vi "Controller FPGA Filter Set Selection.vi"(10 "FPGA Filter Sets":T2(array[cluster]), 11 "selected":i32) -> (2 "Selected FPGA Filter Set":T1)   [LabVIEW 2011, in "Controller VIs.lvlib"]
uses:
  Controller VIs.lvlib
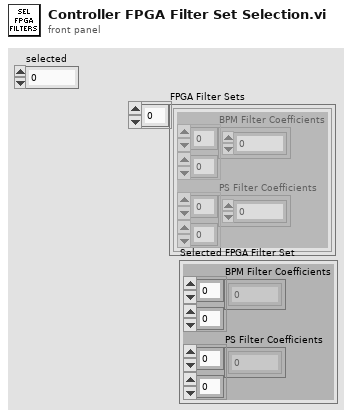
[diagram p1: front panel]
types:
  T1 = cluster{"BPM Filter Coefficients":dbl[][], "PS Filter Coefficients":dbl[][]}
  T2 = cluster{"BPM Filter Coefficients":dbl[][], "PS Filter Coefficients":dbl[][]}[]
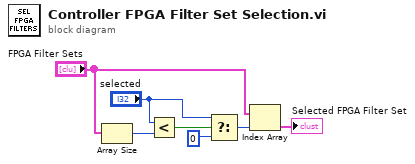
[diagram p0: block diagram]
diagram:
  n1 = Array Size(array="FPGA Filter Sets") -> (size(s)=w4:i32)
  n2 = Less?(x="selected", y=w4) -> (x < y?=w5:bool)
  n3 = Select(t="selected", s=w5, f=0) -> (s? t:f=w2:i32)
  n4 = Index Array(array="FPGA Filter Sets", index=w2) -> (element=→"Selected FPGA Filter Set":T1)
